vi "Simulator.vi"(11 "DataIn":T2) -> (2 "true = ganhou":bool, 3 "Enum":T1)   [LabVIEW 2017]
doc: "SubVI cirada para testar a jogada do PC em todas as posições do tabuleiro, conferindo através do subVI Check se aquela jogada resultaria em uma vitória."
uses:
  controls/DataIn.ctl
  controls/Tabuleiro.ctl
  controls/GameOption.ctl
  controls/TabuleiroCoordenadas.ctl
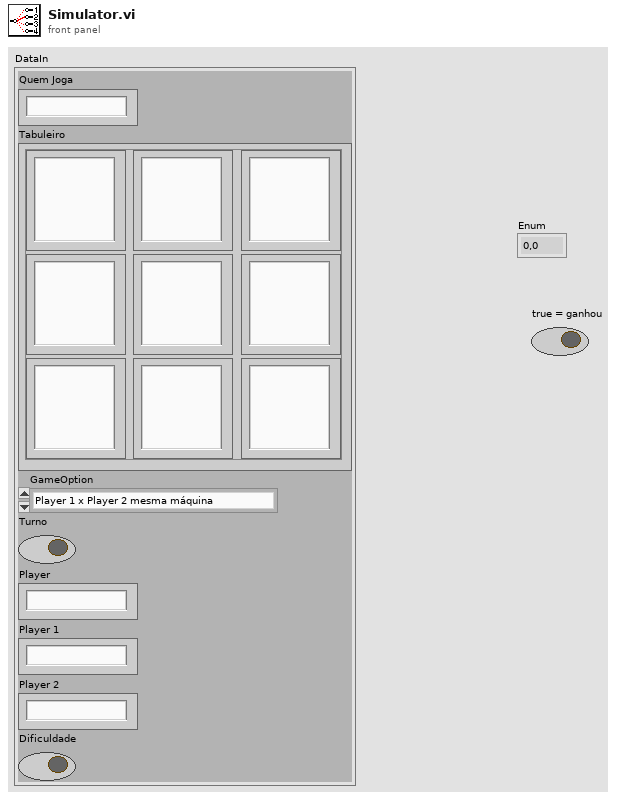
[diagram p1: front panel]
types:
  T1 = typedef "TabuleiroCoordenadas.ctl" = enum16{"0,0", "0,1", "0,2", "1,0", "1,1", "1,2", "2,0", "2,1", "2,2"}
  T2 = typedef "DataIn.ctl" = cluster{"Quem Joga":string, "Tabuleiro":T3, "GameOption":T4, "Turno":bool, "Player":string, "Player 1":string, "Player 2":string, "Dificuldade":bool}
  T3 = typedef "Tabuleiro.ctl" = cluster{"(0,0)":string, "(1,0)":string, "(0,1)":string, "(1,1)":string, "(2,0)":string, "(1,2)":string, "(2,2)":string, "(0,2)":string, "(2,1) ":string}
  T4 = typedef "GameOption.ctl" = enum16{"Player 1 x Player 2 mesma máquina", "Player 1 x Player 2 pela rede", "Player 1 x Computador", "Wait for Event", "Initialize"}
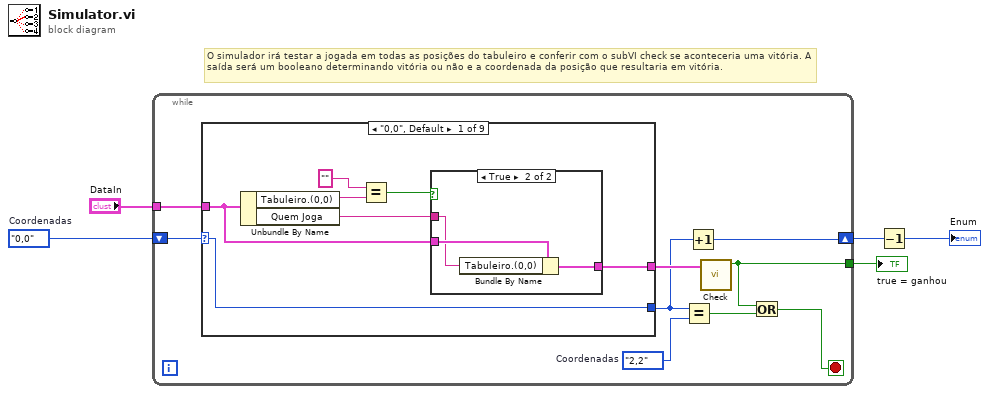
[diagram p0: block diagram]
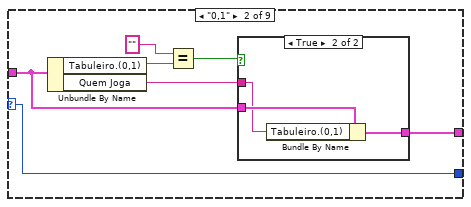
[diagram p3: hidden frame]
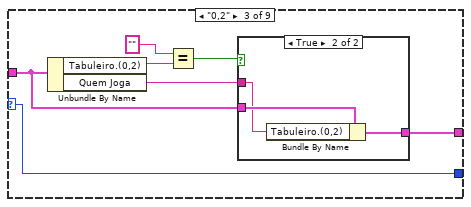
[diagram p5: hidden frame]
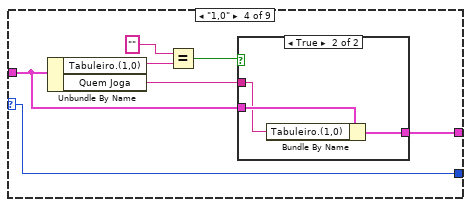
[diagram p7: hidden frame]
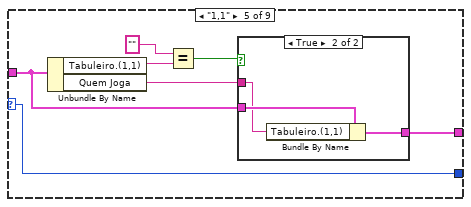
[diagram p9: hidden frame]
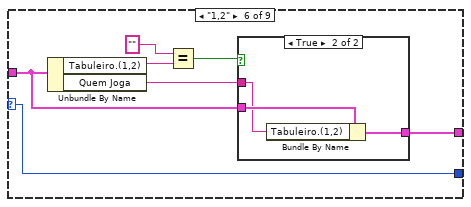
[diagram p11: hidden frame]
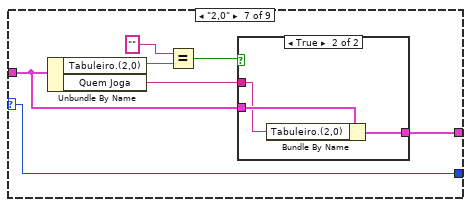
[diagram p13: hidden frame]
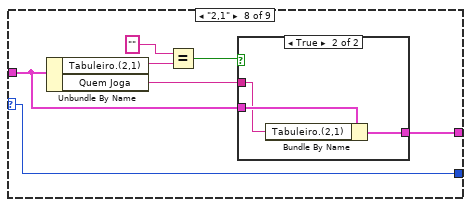
[diagram p15: hidden frame]
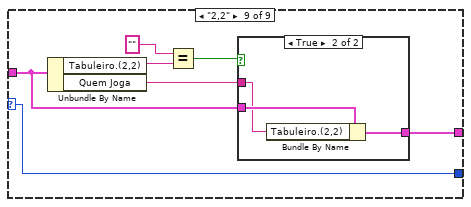
[diagram p17: hidden frame]
diagram:
  w4 = TabuleiroCoordenadas."0,0"  # Coordenadas
  # "O simulador irá testar a jogada em todas as posições do tabuleiro e conferir com o subVI check se aconteceria uma vitória. A saída será um booleano determinando vitória ou não e a coordenada da posição que resultaria em vitória."
  n1 = while {
    tunnel: "DataIn" -> [w14]
    shift-right: [w6] -> w2
    shift-left: w4 -> [w13]
    tunnel: [w8] -> w3
    stop <- w9 stop-if-true
    w11 = TabuleiroCoordenadas."2,2"  # Coordenadas
    n2 = case shown="\"0,0\", Default" w13 {
      selector: w13 -> [w15 w26 w37 w48 w59 w70 w81 w92 w103]
      tunnel: w14 -> [w17 w28 w39 w50 w61 w72 w83 w94 w105]
      tunnel: [w16 w27 w38 w49 w60 w71 w82 w93 w104] -> w12
      tunnel: [w15 w26 w37 w48 w59 w70 w81 w92 w103] -> w7
      frame "0,0", Default {
        n3 = Unbundle By Name(w17) -> ("Tabuleiro.(0,0)"=w21:string, "Quem Joga"=w18:string)
        n4 = Equal?(x="", y=w21) -> (x = y?=w19:bool)
        n5 = case shown="True" w19 {
          tunnel: w18 -> [_ w24]
          tunnel: w17 -> [w22 w25]
          tunnel: [w22 w23] -> w16
          frame False {
          }
          frame True {
            n6 = Bundle By Name(cluster=w25, "Tabuleiro.(0,0)"=w24) -> (w23:T2)
          }
        }
      }
      frame "0,1" {
        n7 = Unbundle By Name(w28) -> ("Tabuleiro.(0,1)"=w32:string, "Quem Joga"=w29:string)
        n8 = Equal?(x="", y=w32) -> (x = y?=w30:bool)
        n9 = case shown="True" w30 {
          tunnel: w29 -> [_ w35]
          tunnel: w28 -> [w33 w36]
          tunnel: [w33 w34] -> w27
          frame False {
          }
          frame True {
            n10 = Bundle By Name(cluster=w36, "Tabuleiro.(0,1)"=w35) -> (w34:T2)
          }
        }
      }
      frame "0,2" {
        n11 = Unbundle By Name(w39) -> ("Tabuleiro.(0,2)"=w43:string, "Quem Joga"=w40:string)
        n12 = Equal?(x="", y=w43) -> (x = y?=w41:bool)
        n13 = case shown="True" w41 {
          tunnel: w40 -> [_ w46]
          tunnel: w39 -> [w44 w47]
          tunnel: [w44 w45] -> w38
          frame False {
          }
          frame True {
            n14 = Bundle By Name(cluster=w47, "Tabuleiro.(0,2)"=w46) -> (w45:T2)
          }
        }
      }
      frame "1,0" {
        n15 = Unbundle By Name(w50) -> ("Tabuleiro.(1,0)"=w54:string, "Quem Joga"=w51:string)
        n16 = Equal?(x="", y=w54) -> (x = y?=w52:bool)
        n17 = case shown="True" w52 {
          tunnel: w51 -> [_ w57]
          tunnel: w50 -> [w55 w58]
          tunnel: [w55 w56] -> w49
          frame False {
          }
          frame True {
            n18 = Bundle By Name(cluster=w58, "Tabuleiro.(1,0)"=w57) -> (w56:T2)
          }
        }
      }
      frame "1,1" {
        n19 = Unbundle By Name(w61) -> ("Tabuleiro.(1,1)"=w65:string, "Quem Joga"=w62:string)
        n20 = Equal?(x="", y=w65) -> (x = y?=w63:bool)
        n21 = case shown="True" w63 {
          tunnel: w62 -> [_ w68]
          tunnel: w61 -> [w66 w69]
          tunnel: [w66 w67] -> w60
          frame False {
          }
          frame True {
            n22 = Bundle By Name(cluster=w69, "Tabuleiro.(1,1)"=w68) -> (w67:T2)
          }
        }
      }
      frame "1,2" {
        n23 = Unbundle By Name(w72) -> ("Tabuleiro.(1,2)"=w76:string, "Quem Joga"=w73:string)
        n24 = Equal?(x="", y=w76) -> (x = y?=w74:bool)
        n25 = case shown="True" w74 {
          tunnel: w73 -> [_ w79]
          tunnel: w72 -> [w77 w80]
          tunnel: [w77 w78] -> w71
          frame False {
          }
          frame True {
            n26 = Bundle By Name(cluster=w80, "Tabuleiro.(1,2)"=w79) -> (w78:T2)
          }
        }
      }
      frame "2,0" {
        n27 = Unbundle By Name(w83) -> ("Tabuleiro.(2,0)"=w87:string, "Quem Joga"=w84:string)
        n28 = Equal?(x="", y=w87) -> (x = y?=w85:bool)
        n29 = case shown="True" w85 {
          tunnel: w84 -> [_ w90]
          tunnel: w83 -> [w88 w91]
          tunnel: [w88 w89] -> w82
          frame False {
          }
          frame True {
            n30 = Bundle By Name(cluster=w91, "Tabuleiro.(2,0)"=w90) -> (w89:T2)
          }
        }
      }
      frame "2,1" {
        n31 = Unbundle By Name(w94) -> ("Tabuleiro.(2,1)"=w98:string, "Quem Joga"=w95:string)
        n32 = Equal?(x="", y=w98) -> (x = y?=w96:bool)
        n33 = case shown="True" w96 {
          tunnel: w95 -> [_ w101]
          tunnel: w94 -> [w99 w102]
          tunnel: [w99 w100] -> w93
          frame False {
          }
          frame True {
            n34 = Bundle By Name(cluster=w102, "Tabuleiro.(2,1)"=w101) -> (w100:T2)
          }
        }
      }
      frame "2,2" {
        n35 = Unbundle By Name(w105) -> ("Tabuleiro.(2,2)"=w109:string, "Quem Joga"=w106:string)
        n36 = Equal?(x="", y=w109) -> (x = y?=w107:bool)
        n37 = case shown="True" w107 {
          tunnel: w106 -> [_ w112]
          tunnel: w105 -> [w110 w113]
          tunnel: [w110 w111] -> w104
          frame False {
          }
          frame True {
            n38 = Bundle By Name(cluster=w113, "Tabuleiro.(2,2)"=w112) -> (w111:T2)
          }
        }
      }
    }
    n39 = Equal?(x=w7, y=w11) -> (x = y?=w10:bool)
    n40 = Increment(x=w7) -> (x+1=w6:T1)
    n41 = call "Check.vi"("DataIn"=w12) -> ("True = Ganhou"=w8:bool)  [unwired: 9 in, 1 out]
    n42 = Or(x=w8, y=w10) -> (x .or. y?=w9:bool)
  }
  "true = ganhou" <- w3
  n43 = Decrement(x=w2) -> (x-1=→"Enum":T1)
